vi "VISP Copy GObjects to Clipboard.vi"(8 "error in (no error)":errorcluster, 10 "GObjects":refnum<vi>[](array[refnum]), 11 "Diagram in":refnum<vi>) -> (0 "error out":errorcluster, 3 "Diagram out":refnum<vi>)   [LabVIEW 2019, in "VI Snippet.lvlib"]
doc: "Makes a selection and copies the <b>GObjects</b> to the clipboard. \n\n<b>Errors:</b>\n1055: \"Object reference invalid\" is raised if the copy failed or <b>GObjects</b> array is empty.\n\nCreated by: Ryan Pacini"
uses:
  VI Snippet.lvlib
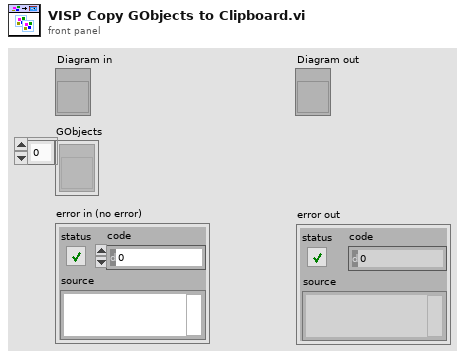
[diagram p1: front panel]
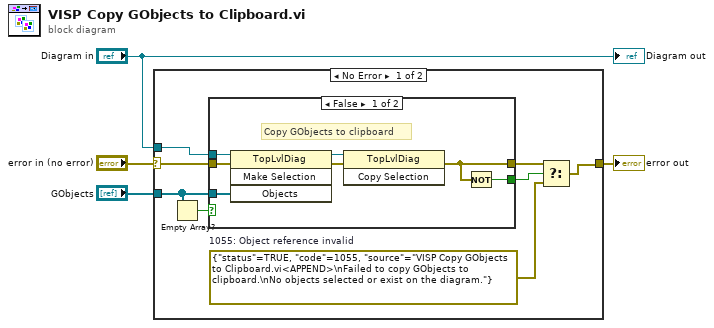
[diagram p0: block diagram]
diagram:
  n1 = case shown="No Error" "error in (no error)" {
    selector: "error in (no error)" -> [w12 w21]
    tunnel: "Diagram in" -> [w10 _]
    tunnel: [w6 w21] -> w3
    tunnel: "GObjects" -> [w11 _]
    frame No Error {
      w8 = errorcluster {"status"=TRUE, "code"=1055, "source"="VISP Copy GObjects to Clipboard.vi<APPEND>\nFailed to copy GObjects to clipboard.\nNo objects selected or exist on the diagram."}  # 1055: Object reference invalid
      n2 = Empty Array?(array=w11) -> (empty?=w5:bool)
      n3 = case shown="False" w5 {
        tunnel: w10 -> [w19 _]
        tunnel: w12 -> [w18 w20]
        tunnel: [w13 w20] -> w7
        tunnel: w11 -> [w15 _]
        tunnel: [w14 _] -> w9
        frame False {
          # "Copy GObjects to clipboard"
          n4 = invoke class="TopLvlDiag" method="Make Selection"(reference=w19, error in=w18, "Objects"=w15) -> (reference out=w16:refnum<vi>, error out=w17:errorcluster)  [unwired: 1 in, 2 out]
          n5 = invoke class="TopLvlDiag" method="Copy Selection"(reference=w16, error in=w17) -> (error out=w13:errorcluster)  [unwired: 1 in, 2 out]
          n6 = Not(x=w13) -> (.not. x?=w14:bool)
        }
        frame True {
        }
      }
      n7 = Select(t=w7, s=w9, f=w8) -> (s? t:f=w6:errorcluster)
    }
    frame Error {
    }
  }
  "error out" <- w3
  "Diagram out" <- "Diagram in"
